vi "GetStreamMode.vi"(7 "Timeout (ms)":u32=2000, 8 "Error In":errorcluster, 11 "Sierra M100 In":refnum<visa-resource-name>) -> (0 "Error Out":errorcluster, 3 "Sierra M100 Out":refnum<visa-resource-name>)   [LabVIEW 2012, in "Sierra-M100.lvlib"]
doc: "This VI gets the streaming mode."
uses:
  Sierra-M100.lvlib
  Controls/StreamMode.ctl
panel:
  out "Mode":T1
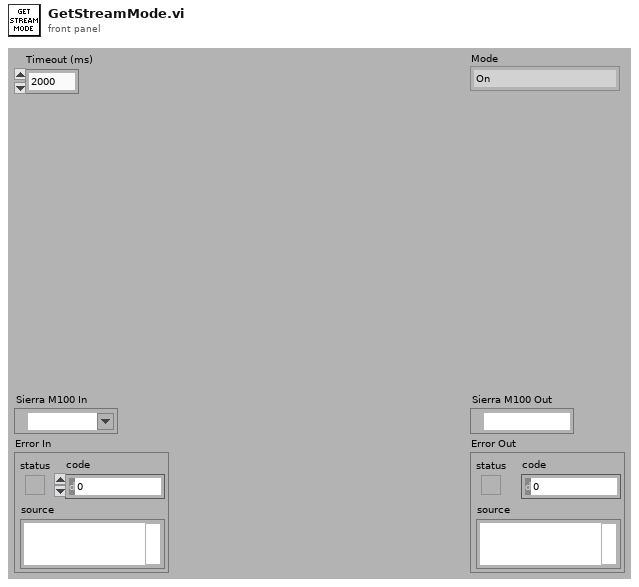
[diagram p1: front panel]
types:
  T1 = typedef "Sierra-M100.lvlib/StreamMode.ctl" = enum16{"On", "Off", "Echo"}
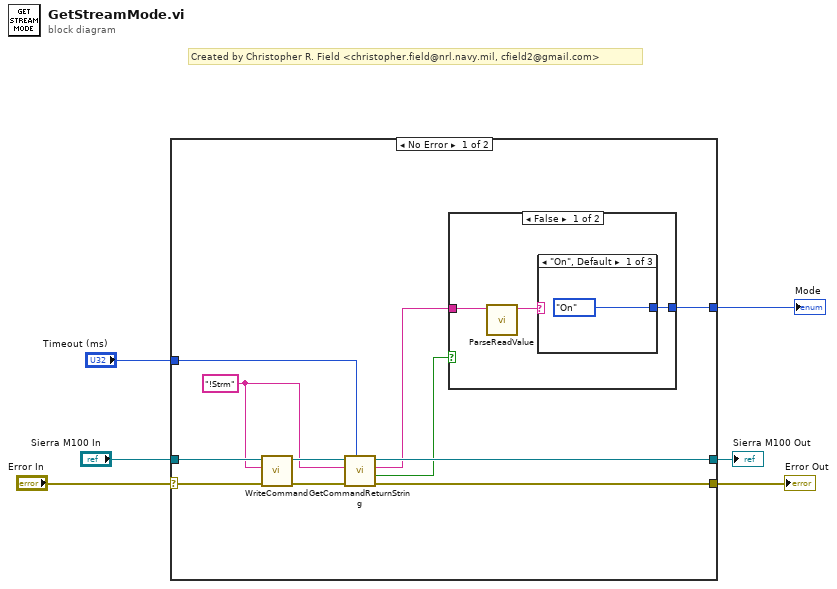
[diagram p0: block diagram]
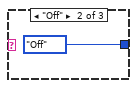
[diagram p2: hidden frame]
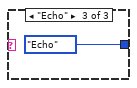
[diagram p3: hidden frame]
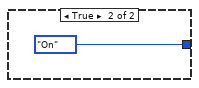
[diagram p4: hidden frame]
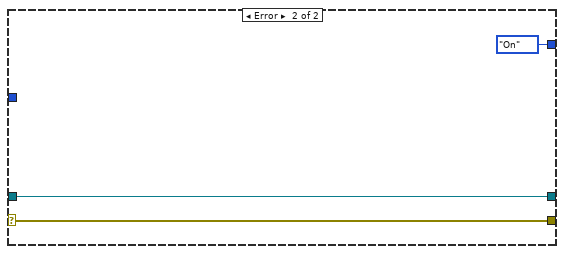
[diagram p5: hidden frame]
diagram:
  # "Created by Christopher R. Field <christopher.field@nrl.navy.mil, cfield2@gmail.com>"
  n1 = case shown="No Error" "Error In" {
    selector: "Error In" -> [w7 w26]
    tunnel: "Sierra M100 In" -> [w17 w27]
    tunnel: "Timeout (ms)" -> [w13 _]
    tunnel: [w12 w27] -> w4
    tunnel: [w11 w26] -> w3
    tunnel: [w8 enum16{"On", "Off", "Echo"}."On" ("Mode")] -> w2
    frame No Error {
      w14 = "!Strm"
      n2 = call "WriteCommand.vi"("Error In"=w7, "Command"=w14, "Smart Trak 2 In"=w17) -> ("Error Out"=w15:errorcluster, "Smart Trak 2 Out"=w16:refnum<visa-resource-name>)  [unwired: 5 in, 2 out]
      n3 = call "GetCommandReturnString.vi"("Timeout (ms)"=w13, "Error In"=w15, "Command"=w14, "Smart Trak 2 In"=w16) -> ("Error Out"=w11:errorcluster, "Timeout?"=w10:bool, "Return String"=w9:string, "Smart Trak 2 Out"=w12:refnum<visa-resource-name>)  [unwired: 4 in]
      n4 = case shown="False" w10 {
        tunnel: [w20 enum16{"On", "Off", "Echo"}."On" ("Mode")] -> w8
        tunnel: w9 -> [w18 _]
        frame False {
          n5 = call "ParseReadValue.vi"("Read Buffer"=w18) -> ("Value"=w19:string)  [unwired: 10 in]
          n6 = case shown="\"On\", Default" w19 {
            tunnel: [enum16{"On", "Off", "Echo"}."On" ("Mode") enum16{"On", "Off", "Echo"}."Off" ("Mode") enum16{"On", "Off", "Echo"}."Echo" ("Mode")] -> w20
            frame "On", Default {
            }
            frame "Off" {
            }
            frame "Echo" {
            }
          }
        }
        frame True {
        }
      }
    }
    frame Error {
    }
  }
  "Sierra M100 Out" <- w4
  "Error Out" <- w3
  "Mode" <- w2
